vi "deleteEvent.vi"(8 "error in (no error)":errorcluster, 9 "selectedEvent":i32, 10 "Enum":enum16{"Update_dt", "Update_Time"}(ring), 11 "ScriptEventList in":refnum<class "ScriptEventList.lvclass">) -> (0 "error out":errorcluster, 3 "ScriptEventList out":refnum<class "ScriptEventList.lvclass">)   [LabVIEW 2009, in "Tools.lvlib" / "Scripting.lvlib" / "ScriptEventList.lvclass"]
uses:
  ScriptEventList.lvclass
  ScriptEventList.lvclass/ScriptEventList.ctl
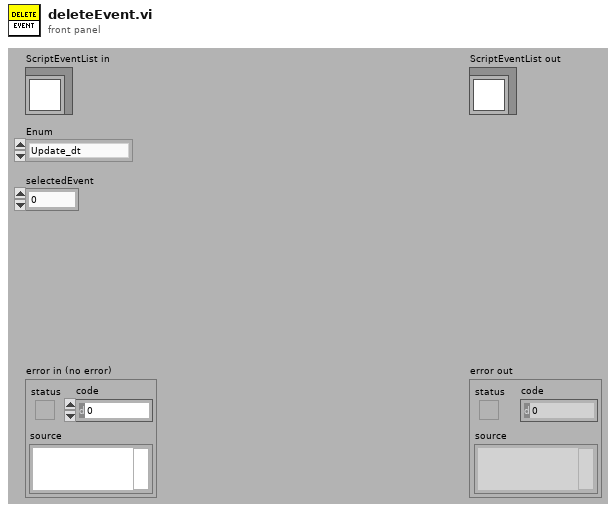
[diagram p1: front panel]
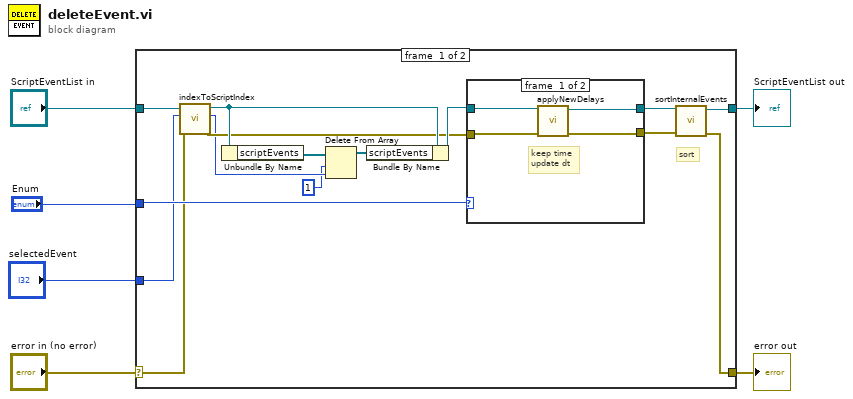
[diagram p0: block diagram]
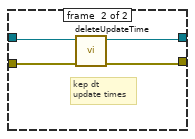
[diagram p2: hidden frame]
diagram:
  n1 = case shown="No Error" "error in (no error)" {
    selector: "error in (no error)" -> [w14 w31]
    tunnel: [w18 w31] -> w5
    tunnel: [w17 w30] -> w3
    tunnel: "ScriptEventList in" -> [w16 w30]
    tunnel: "Enum" -> [w21 _]
    tunnel: "selectedEvent" -> [w15 _]
    frame #0 {
      # "sort"
      n2 = call "indexToScriptIndex.vi"("error in (no error)"=w14, "sequencedIndex"=w15, "ScriptEventList in"=w16) -> ("error out"=w9:errorcluster, "indexScriptEvent"=w8:i32, "ScriptEventList out"=w11:refnum<class "ScriptEventList.lvclass">)  [unwired: 6 in]
      n3 = Unbundle By Name(w11) -> ("scriptEvents"=w13:refnum<class "ScriptEvent.lvclass">[])
      n4 = Delete From Array(array=w13, length=1, index=w8) -> (array with subset deleted=w12:refnum<class "ScriptEvent.lvclass">[])  [unwired: 1 out]
      n5 = Bundle By Name(cluster=w11, "scriptEvents"=w12) -> (w10:refnum<class "ScriptEventList.lvclass">)
      n6 = case shown="\"Update_dt\", Default" w21 {
        tunnel: w10 -> [w25 w29]
        tunnel: [w24 w26] -> w20
        tunnel: w9 -> [w22 w28]
        tunnel: [w23 w27] -> w19
        frame #0 {
          # "keep time\nupdate dt"
          n7 = call "applyNewDelays.vi"("error in (no error)"=w22, "ScriptEventList in"=w25) -> ("error out"=w23:errorcluster, "ScriptEventList out"=w24:refnum<class "ScriptEventList.lvclass">)  [unwired: 8 in]
        }
        frame #1 {
          # "kep dt\nupdate times"
          n8 = call "deleteUpdateTime.vi"("error in (no error)"=w28, "ScriptEventList in"=w29) -> ("error out"=w27:errorcluster, "ScriptEventList out"=w26:refnum<class "ScriptEventList.lvclass">)  [unwired: 8 in]
        }
      }
      n9 = call "sortInternalEvents.vi"("error in (no error)"=w19, "ScriptEventList in"=w20) -> ("error out"=w18:errorcluster, "ScriptEventList out"=w17:refnum<class "ScriptEventList.lvclass">)  [unwired: 8 in]
    }
    frame #1 {
    }
  }
  "error out" <- w5
  "ScriptEventList out" <- w3
